vi "FTW-Crypto-HMAC-Hasher.vi"(0 "Data":string="Data to encrypt!", 5 "Key":string, 7 "Algorithm":enum16{"SHA512", "SHA256", "SHA1", "MD5"}(ring), 9 "Hash Encoding":enum16{"No encoding", "Base64", "ASCII Hex"}(ring)=enum."ASCII Hex", 11 "error in":errorcluster) -> (4 "Hash out":string, 15 "error out":errorcluster)   [LabVIEW 2012]
panel:
  out "Hash Length":i32
  # "Inputs"
  # "Outputs"
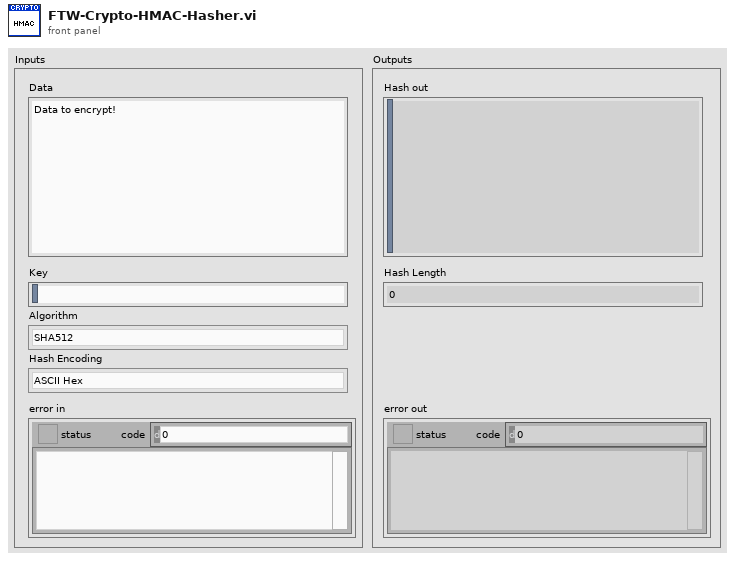
[diagram p1: front panel]
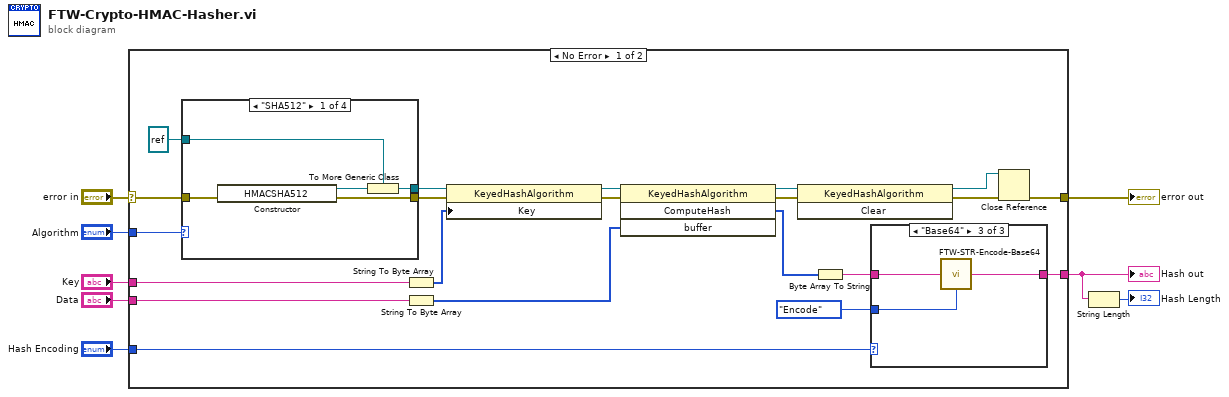
[diagram p0: block diagram]
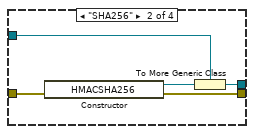
[diagram p2: hidden frame]
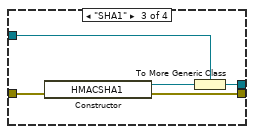
[diagram p3: hidden frame]
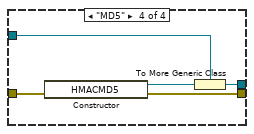
[diagram p4: hidden frame]
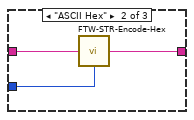
[diagram p6: hidden frame]
diagram:
  n1 = case shown="No Error" "error in" {
    selector: "error in" -> [w28 w57]
    tunnel: "Data" -> [w11 _]
    tunnel: [w19 _] -> w3
    tunnel: "Key" -> [w10 _]
    tunnel: [w27 w57] -> w5
    tunnel: "Hash Encoding" -> [w21 _]
    tunnel: "Algorithm" -> [w17 _]
    frame No Error {
      n2 = case shown="\"SHA512\"" w17 {
        tunnel: [w34 w39 w44 w49] -> w13
        tunnel: w28 -> [w33 w38 w43 w48]
        tunnel: [w31 w36 w41 w46] -> w15
        tunnel: refnum<k24> refnum (".NET Refnum") -> [w30 w35 w40 w45]
        frame "SHA512" {
          n3 = constructor class="HMACSHA512"(error in=w33) -> (reference out=w32:refnum<k24>, error out=w34:errorcluster)  [unwired: 2 in, 1 out]
          n4 = To More Generic Class(target class=w30, reference=w32) -> (generic class reference=w31:refnum<k24>)
        }
        frame "SHA256" {
          n5 = constructor class="HMACSHA256"(error in=w38) -> (reference out=w37:refnum<k24>, error out=w39:errorcluster)  [unwired: 2 in, 1 out]
          n6 = To More Generic Class(target class=w35, reference=w37) -> (generic class reference=w36:refnum<k24>)
        }
        frame "SHA1" {
          n7 = constructor class="HMACSHA1"(error in=w43) -> (reference out=w42:refnum<k24>, error out=w44:errorcluster)  [unwired: 2 in, 1 out]
          n8 = To More Generic Class(target class=w40, reference=w42) -> (generic class reference=w41:refnum<k24>)
        }
        frame "MD5" {
          n9 = constructor class="HMACMD5"(error in=w48) -> (reference out=w47:refnum<k24>, error out=w49:errorcluster)  [unwired: 2 in, 1 out]
          n10 = To More Generic Class(target class=w45, reference=w47) -> (generic class reference=w46:refnum<k24>)
        }
      }
      n11 = String To Byte Array(string=w10) -> (unsigned byte array=w9:u8[])
      n12 = String To Byte Array(string=w11) -> (unsigned byte array=w29:u8[])
      n13 = property class="KeyedHashAlgorithm"(reference=w15, error in=w13, "Key"=w9) -> (reference out=w14:refnum<k24>, error out=w12:errorcluster)
      n14 = invoke class="KeyedHashAlgorithm" method="ComputeHash"(reference=w14, error in=w12, "buffer"=w29) -> (reference out=w25:refnum<k24>, error out=w24:errorcluster, "ComputeHash"=w26:u8[])  [unwired: 1 in, 1 out]
      n15 = invoke class="KeyedHashAlgorithm" method="Clear"(reference=w25, error in=w24) -> (reference out=w22:refnum<k24>, error out=w23:errorcluster)  [unwired: 1 in, 1 out]
      n16 = Byte Array To String(unsigned byte array=w26) -> (string=w20:string)
      n17 = case shown="\"Base64\"" w21 {
        tunnel: w20 -> [w50 w53 w56]
        tunnel: [w50 w51 w55] -> w19
        tunnel: enum16{"Encode", "Decode"}."Encode" ("Direction") -> [_ w52 w54]
        frame "No encoding" {
        }
        frame "ASCII Hex" {
          n18 = call "FTW-STR-Encode-Hex.vi"("Input"=w53, "Direction"=w52) -> ("Output"=w51:string)
        }
        frame "Base64" {
          n19 = call "FTW-STR-Encode-Base64.vi"("Input"=w56, "Direction"=w54) -> ("Output"=w55:string)
        }
      }
      n20 = Close Reference(reference=w22, error in (no error)=w23) -> (error out=w27:errorcluster)
    }
    frame Error {
    }
  }
  "Hash out" <- w3
  "error out" <- w5
  n21 = String Length(string=w3) -> (length=→"Hash Length":i32)
